vi "Opgave 1 Arealberegning.vi"(10 "beregningstype":enum16{"Omkreds", "Areal"}(ring)=enum."Areal", 11 "Højde":dbl=2.0) -> (3 "Resultat":dbl)   [LabVIEW 2019]
doc: "Skrevet til test af autoretter"
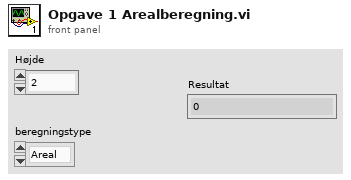
[diagram p1: front panel]
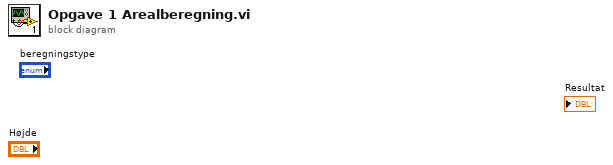
[diagram p0: block diagram]
diagram:
